vi "LoadPodTurretData.vi"(9 "Pod Number":i32, 10 "Pod Configuration in":T2, 11 "Config file Refnum in":T1) -> (2 "Pod Configuration out":T2, 3 "Config file Refnum out":T1)   [LabVIEW 2014]
uses:
  <vilib>/Utility/config.llb/Config Data RefNum.ctl
  <vilib>/Utility/config.llb/Read Key (I32).vi
  <vilib>/Utility/config.llb/Write Key (I32).vi
  <vilib>/Utility/config.llb/Read Key (Boolean).vi
  <vilib>/Utility/config.llb/Write Key (Boolean).vi
  <vilib>/Utility/config.llb/Read Key (Double).vi
  <vilib>/Utility/config.llb/Write Key (Double).vi
  <vilib>/Utility/config.llb/Read Key (String).vi
  <vilib>/Utility/config.llb/Write Key (String).vi
  <vilib>/Utility/config.llb/NI_LVConfig.lvlib
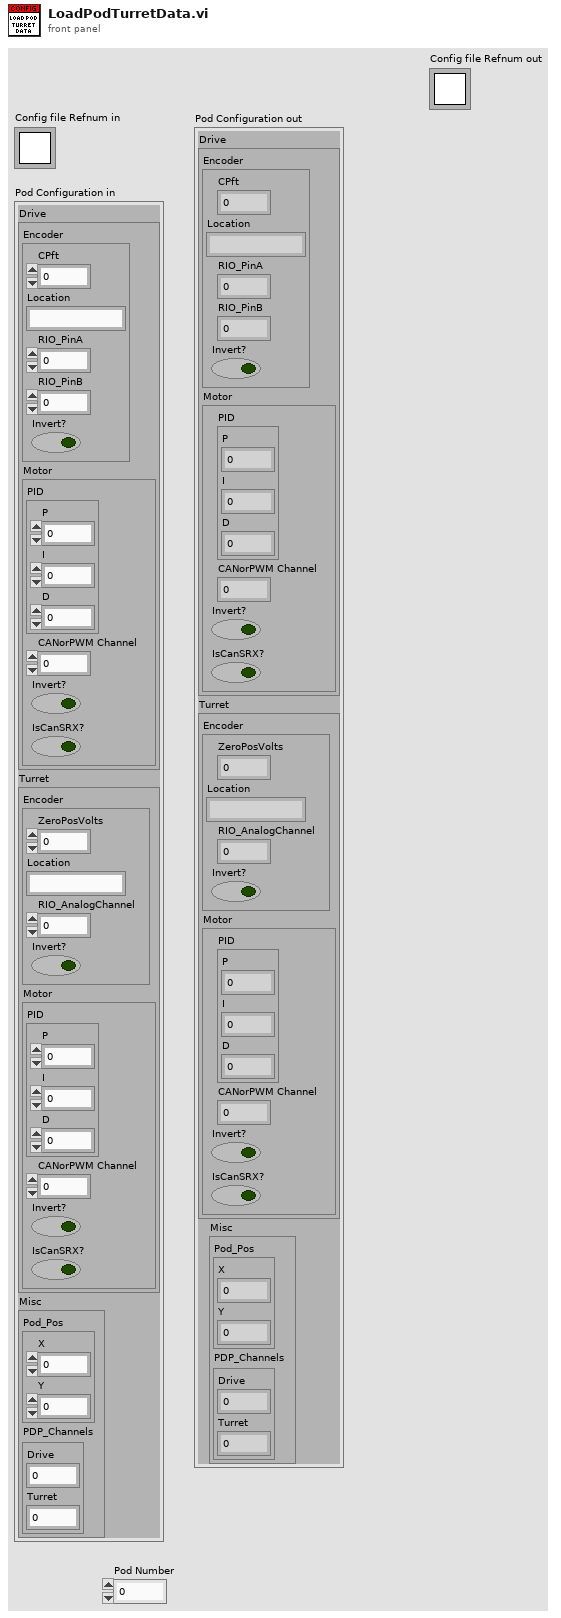
[diagram p1: front panel]
types:
  T1 = typedef "NI_LVConfig.lvlib/Config Data RefNum.ctl" = refnum<k1>
  T2 = cluster{"Drive":cluster{"Encoder":cluster{"CPft":dbl, "Location":string, "RIO_PinA":i32, "RIO_PinB":i32, "Invert?":bool}, "Motor":cluster{"PID":cluster{"P":dbl, "I":dbl, "D":dbl}, "CANorPWM Channel":i32, "Invert?":bool, "IsCanSRX?":bool}}, "Turret":cluster{"Encoder":cluster{"ZeroPosVolts":dbl, "Location":string, "RIO_AnalogChannel":i32, "Invert?":bool}, "Motor":cluster{"PID":cluster{"P":dbl, "I":dbl, "D":dbl}, "CANorPWM Channel":i32, "Invert?":bool, "IsCanSRX?":bool}}, "Misc":cluster{"Pod_Pos":cluster{"X":dbl, "Y":dbl}, "PDP_Channels":cluster{"Drive":i32, "Turret":i32}}}
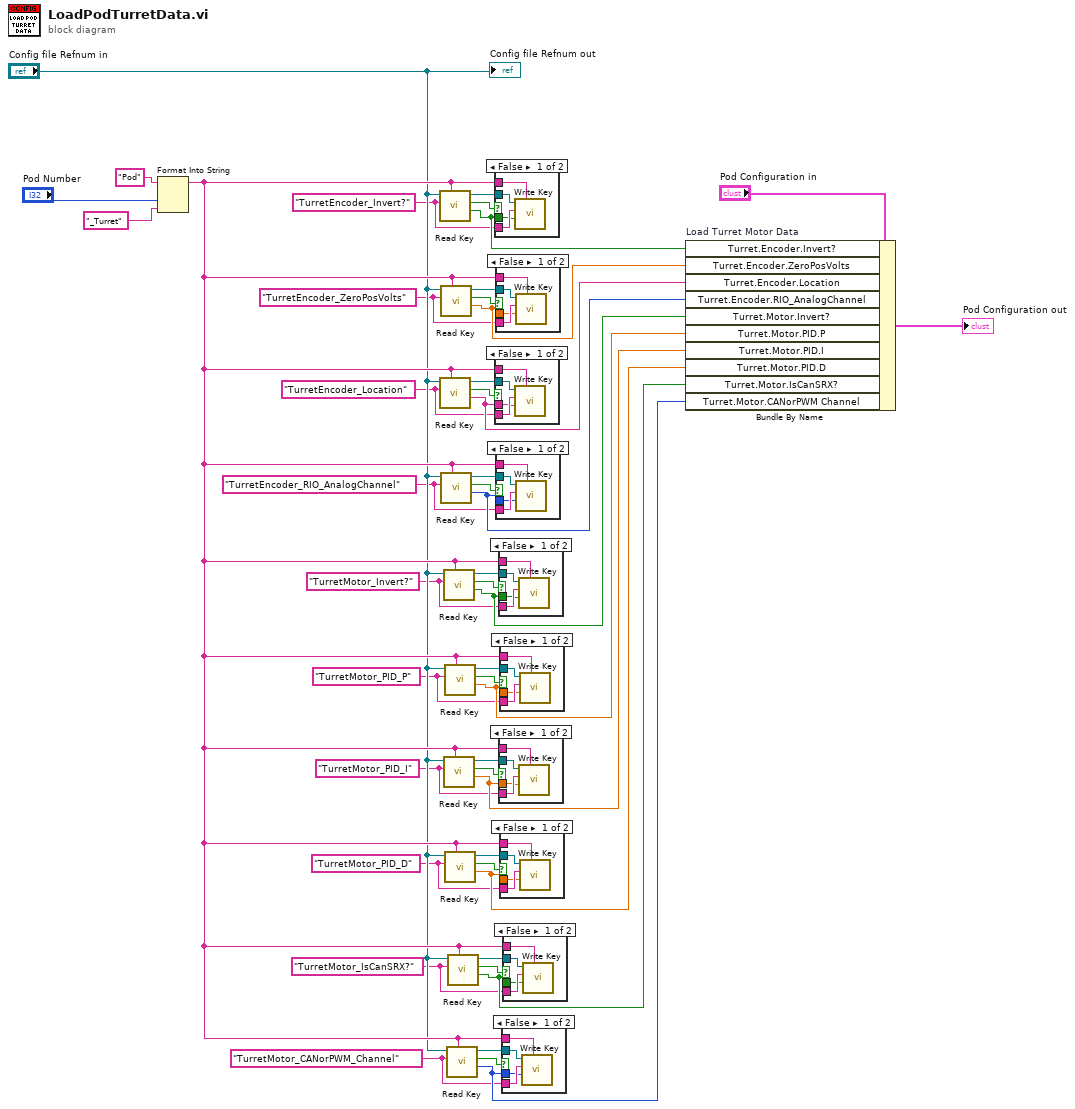
[diagram p0: block diagram]
diagram:
  w40 = "TurretMotor_CANorPWM_Channel" ("string")
  w37 = "TurretMotor_IsCanSRX?" ("string")
  w24 = "TurretMotor_PID_D" ("string")
  w23 = "TurretMotor_PID_I" ("string")
  w29 = "TurretMotor_PID_P" ("string")
  w30 = "TurretMotor_Invert?" ("string")
  w15 = "TurretEncoder_RIO_AnalogChannel" ("string")
  w16 = "TurretEncoder_Location" ("string")
  w8 = "TurretEncoder_ZeroPosVolts" ("string")
  w7 = "TurretEncoder_Invert?" ("string")
  n1 = Format Into String(initial string="Pod", "Pod Number", "_Turret") -> (resulting string=w46:string)  [unwired: 2 in, 1 out]
  n2 = call-poly <vilib>:"Read Key.vi"("section"=w46, "key"=w7, "refnum"="Config file Refnum in") -> ("value"=w11:bool, "found?"=w5:bool, "refnum out"=w6:T1)  [unwired: 5 in, 1 out]
  n3 = call-poly <vilib>:"Read Key.vi"("section"=w46, "key"=w16, "refnum"="Config file Refnum in") -> ("value"=w19:string, "found?"=w18:bool, "refnum out"=w17:T1)  [unwired: 5 in, 1 out]
  n4 = call-poly <vilib>:"Read Key.vi"("section"=w46, "key"=w8, "refnum"="Config file Refnum in") -> ("value"=w12:dbl, "found?"=w10:bool, "refnum out"=w9:T1)  [unwired: 5 in, 1 out]
  n5 = call-poly <vilib>:"Read Key.vi"("section"=w46, "key"=w15, "refnum"="Config file Refnum in") -> ("value"=w20:i32, "found?"=w13:bool, "refnum out"=w14:T1)  [unwired: 5 in, 1 out]
  n6 = call-poly <vilib>:"Read Key.vi"("section"=w46, "key"=w30, "refnum"="Config file Refnum in") -> ("value"=w33:bool, "found?"=w32:bool, "refnum out"=w31:T1)  [unwired: 5 in, 1 out]
  n7 = call-poly <vilib>:"Read Key.vi"("section"=w46, "key"=w23, "refnum"="Config file Refnum in") -> ("value"=w35:dbl, "found?"=w21:bool, "refnum out"=w22:T1)  [unwired: 5 in, 1 out]
  n8 = call-poly <vilib>:"Read Key.vi"("section"=w46, "key"=w29, "refnum"="Config file Refnum in") -> ("value"=w34:dbl, "found?"=w27:bool, "refnum out"=w28:T1)  [unwired: 5 in, 1 out]
  n9 = call-poly <vilib>:"Read Key.vi"("section"=w46, "key"=w24, "refnum"="Config file Refnum in") -> ("value"=w36:dbl, "found?"=w26:bool, "refnum out"=w25:T1)  [unwired: 5 in, 1 out]
  n10 = call-poly <vilib>:"Read Key.vi"("section"=w46, "key"=w40, "refnum"="Config file Refnum in") -> ("value"=w45:i32, "found?"=w42:bool, "refnum out"=w41:T1)  [unwired: 5 in, 1 out]
  n11 = call-poly <vilib>:"Read Key.vi"("section"=w46, "key"=w37, "refnum"="Config file Refnum in") -> ("value"=w44:bool, "found?"=w39:bool, "refnum out"=w38:T1)  [unwired: 5 in, 1 out]
  n12 = case shown="False" w5 {
    tunnel: w6 -> [w51 _]
    tunnel: w46 -> [w50 _]
    tunnel: w7 -> [w49 _]
    tunnel: w11 -> [w48 _]
    frame False {
      n13 = call-poly <vilib>:"Write Key.vi"("section"=w50, "value"=w48, "key"=w49, "refnum"=w51) -> ()  [unwired: 5 in, 3 out]
    }
    frame True {
    }
  }
  n14 = case shown="False" w18 {
    tunnel: w17 -> [w55 _]
    tunnel: w46 -> [w54 _]
    tunnel: w16 -> [w53 _]
    tunnel: w19 -> [w52 _]
    frame False {
      n15 = call-poly <vilib>:"Write Key.vi"("section"=w54, "value"=w52, "key"=w53, "refnum"=w55) -> ()  [unwired: 5 in, 3 out]
    }
    frame True {
    }
  }
  n16 = case shown="False" w10 {
    tunnel: w9 -> [w59 _]
    tunnel: w46 -> [w58 _]
    tunnel: w8 -> [w57 _]
    tunnel: w12 -> [w56 _]
    frame False {
      n17 = call-poly <vilib>:"Write Key.vi"("section"=w58, "value"=w56, "key"=w57, "refnum"=w59) -> ()  [unwired: 5 in, 3 out]
    }
    frame True {
    }
  }
  n18 = case shown="False" w13 {
    tunnel: w14 -> [w63 _]
    tunnel: w46 -> [w62 _]
    tunnel: w15 -> [w61 _]
    tunnel: w20 -> [w60 _]
    frame False {
      n19 = call-poly <vilib>:"Write Key.vi"("section"=w62, "value"=w60, "key"=w61, "refnum"=w63) -> ()  [unwired: 5 in, 3 out]
    }
    frame True {
    }
  }
  n20 = case shown="False" w32 {
    tunnel: w31 -> [w67 _]
    tunnel: w46 -> [w66 _]
    tunnel: w30 -> [w65 _]
    tunnel: w33 -> [w64 _]
    frame False {
      n21 = call-poly <vilib>:"Write Key.vi"("section"=w66, "value"=w64, "key"=w65, "refnum"=w67) -> ()  [unwired: 5 in, 3 out]
    }
    frame True {
    }
  }
  n22 = case shown="False" w21 {
    tunnel: w22 -> [w71 _]
    tunnel: w46 -> [w70 _]
    tunnel: w23 -> [w69 _]
    tunnel: w35 -> [w68 _]
    frame False {
      n23 = call-poly <vilib>:"Write Key.vi"("section"=w70, "value"=w68, "key"=w69, "refnum"=w71) -> ()  [unwired: 5 in, 3 out]
    }
    frame True {
    }
  }
  n24 = case shown="False" w27 {
    tunnel: w28 -> [w75 _]
    tunnel: w46 -> [w74 _]
    tunnel: w29 -> [w73 _]
    tunnel: w34 -> [w72 _]
    frame False {
      n25 = call-poly <vilib>:"Write Key.vi"("section"=w74, "value"=w72, "key"=w73, "refnum"=w75) -> ()  [unwired: 5 in, 3 out]
    }
    frame True {
    }
  }
  n26 = case shown="False" w26 {
    tunnel: w25 -> [w79 _]
    tunnel: w46 -> [w78 _]
    tunnel: w24 -> [w77 _]
    tunnel: w36 -> [w76 _]
    frame False {
      n27 = call-poly <vilib>:"Write Key.vi"("section"=w78, "value"=w76, "key"=w77, "refnum"=w79) -> ()  [unwired: 5 in, 3 out]
    }
    frame True {
    }
  }
  n28 = case shown="False" w42 {
    tunnel: w41 -> [w83 _]
    tunnel: w46 -> [w82 _]
    tunnel: w40 -> [w81 _]
    tunnel: w45 -> [w80 _]
    frame False {
      n29 = call-poly <vilib>:"Write Key.vi"("section"=w82, "value"=w80, "key"=w81, "refnum"=w83) -> ()  [unwired: 5 in, 3 out]
    }
    frame True {
    }
  }
  n30 = case shown="False" w39 {
    tunnel: w38 -> [w87 _]
    tunnel: w46 -> [w86 _]
    tunnel: w37 -> [w85 _]
    tunnel: w44 -> [w84 _]
    frame False {
      n31 = call-poly <vilib>:"Write Key.vi"("section"=w86, "value"=w84, "key"=w85, "refnum"=w87) -> ()  [unwired: 5 in, 3 out]
    }
    frame True {
    }
  }
  n32 = Bundle By Name "Load Turret Motor Data"(cluster="Pod Configuration in", "Turret.Encoder.Invert?"=w11, "Turret.Encoder.ZeroPosVolts"=w12, "Turret.Encoder.Location"=w19, "Turret.Encoder.RIO_AnalogChannel"=w20, "Turret.Motor.Invert?"=w33, "Turret.Motor.PID.P"=w34, "Turret.Motor.PID.I"=w35, "Turret.Motor.PID.D"=w36, "Turret.Motor.IsCanSRX?"=w44, "Turret.Motor.CANorPWM Channel"=w45) -> (→"Pod Configuration out":T2)
  "Config file Refnum out" <- "Config file Refnum in"
